vi "CPU_MEM_Kernal_ROM_RE.vi"(11 "address":u16 format="%.0x") -> (2 "value out":u8 format="%02x")   [LabVIEW 2018]
uses:
  CPU_MEM_references.vi
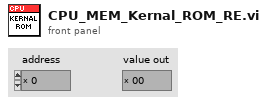
[diagram p1: front panel]
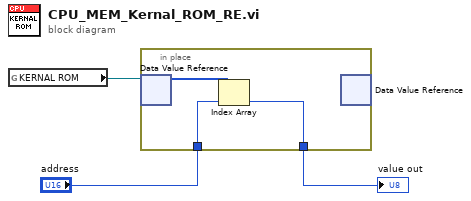
[diagram p0: block diagram]
diagram:
  n1 = global read "CPU_MEM_references.vi" "KERNAL ROM"() -> (w1:refnum<data-value>)
  n2 = in-place {
    in-place-border: "address" -> [w6]
    in-place-border: [w5] -> w2
    n3 = in-place-dvr #1(w1) -> (w4:u8[])  [unwired: 1 out]
    n4 = Index Array(array=w4, index=w6) -> (element=w5:u8)
    n5 = in-place-dvr #1() -> ()  [unwired: 1 in, 2 out]
  }
  "value out" <- w2
